vi "Move Existing Config Files.vi"   [LabVIEW 2016, in "Control Experiment.lvclass"]
uses:
  Control Experiment.lvclass
  <vilib>/Utility/sysdir.llb/System Directory Type.ctl
types:
  T1 = typedef "System Directory Type.ctl" = i32
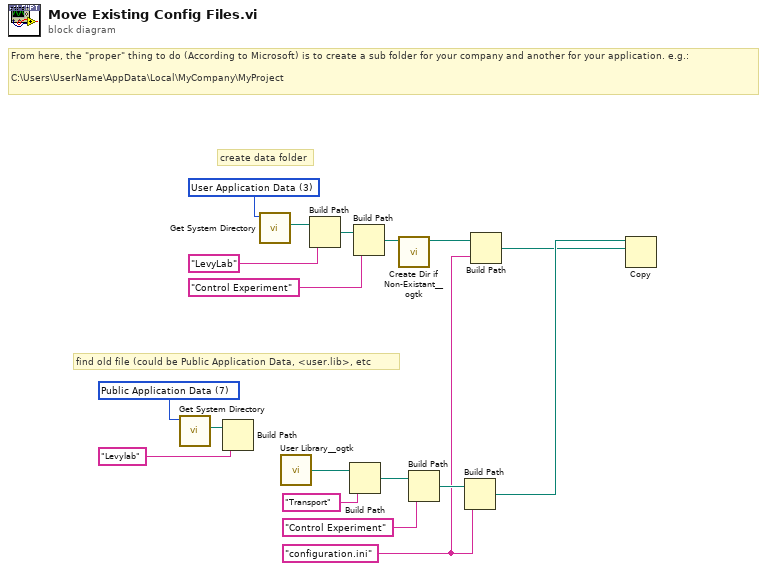
[diagram p0: block diagram]
diagram:
  w15 = T1 3 items=["User Home"=0, "User Desktop"=1, "User Documents"=2, "User Application Data"=3, "User Preferences"=4, "User Temporary"=5, "Public Documents"=6, "Public Application Data"=7, "Public Preferences"=8, "Public Cache"=13, "System Core Libraries"=9, "System Installed Libraries"=10, "Application Files"=11, "Boot Volume Root"=12] ("system directory type")
  w2 = "configuration.ini" ("name or relative path")
  w18 = T1 7 items=["User Home"=0, "User Desktop"=1, "User Documents"=2, "User Application Data"=3, "User Preferences"=4, "User Temporary"=5, "Public Documents"=6, "Public Application Data"=7, "Public Preferences"=8, "Public Cache"=13, "System Core Libraries"=9, "System Installed Libraries"=10, "Application Files"=11, "Boot Volume Root"=12] ("system directory type")
  # "find old file (could be Public Application Data, <user.lib>, etc"
  # "From here, the \"proper\" thing to do (According to Microsoft) is to create a sub folder for your company and another for your application. e.g.:\n\nC:\\Users\\UserName\\AppData\\Local\\MyCompany\\MyProject"
  # "create data folder"
  n1 = call <vilib>:"Get System Directory.vi"("system directory type"=w18) -> ("system directory"=w16:path)  [unwired: 10 in]
  n2 = Build Path(base path=w16, name or relative path="Levylab") -> ()  [unwired: 1 out]
  n3 = call <vilib>:"Get System Directory.vi"("system directory type"=w15) -> ("system directory"=w14:path)  [unwired: 10 in]
  n4 = call <userlib>:"User Library__ogtk.vi"() -> ("User Library (+ Relative)"=w6:path)  [unwired: 1 in]
  n5 = Build Path(base path=w14, name or relative path="LevyLab") -> (appended path=w11:path)
  n6 = Build Path(base path=w6, name or relative path="Transport") -> (appended path=w12:path)
  n7 = Build Path(base path=w11, name or relative path="Control Experiment") -> (appended path=w9:path)
  n8 = call <userlib>:"Create Dir if Non-Existant__ogtk.vi"("Directory Path"=w9) -> ("dup Directory Path"=w3:path)  [unwired: 8 in, 2 out]
  n9 = Build Path(base path=w12, name or relative path="Control Experiment") -> (appended path=w8:path)
  n10 = Build Path(base path=w8, name or relative path=w2) -> (appended path=w4:path)
  n11 = Build Path(base path=w3, name or relative path=w2) -> (appended path=w1:path)
  n12 = Copy(10:w1, 11:w4) -> ()  [unwired: 3 in, 3 out]
